vi "CmdWriter with Context.vi"() -> ()   [LabVIEW 2020]
doc: "Copyright © 2008 - 2024 VI Technologies B.V. \nALL RIGHTS RESERVED"
uses:
  <vilib>/dex/Stream Element Allocation Mode.ctl
  SuperNS/SuperNS.lvclass
  MsgData/MsgData.lvclass
panel:
  in  "Connection Config":T2={"BufferSize (100)"=100, "Connection Lost Timeout (2000 ms)"=2000, "Element Allocation Mode"=0, "Low latency mode"=enum."None (High througput mode)", "BG ConnCheck/Read period (200 ms)"=200, "OpenProcessWindow"=TRUE} {"Element Allocation Mode" items=["allocate as needed", "pre-allocate"]}
  out "error out":errorcluster
  in  "Remote EP Config":T3={"IP"="localhost", "Context"="ReadTestEnv", "Name"="ReaderTest"}
  in  "Local EP Config":cluster{"Context":string, "Name":string}={"Context"="WriteTestEnv", "Name"="WriterTest"}
  in  "Send":bool
  in  "Message":string
  # "Copyright (c) 2024, VI Technologies B.V.\nAll rights reserved.\n\nRedistribution and use in source and binary forms, with or without modification, are permitted provided that \nthe following conditions are met:\n\n * Redistributions of source code must retain the above copyright notice, this list of conditions and the \nfollowing disclaimer.\n * Redistributions in binary form must reproduce the above copyright notice, this list of conditions and the \nfollowing disclaimer in the documentation and/or other materials provided with the distribution.\n * Neither the name of VI Technologies B.V. nor the names of its contributors may be used to endorse or \npromote products derived from this software without specific prior written permission.\n\nTHIS SOFTWARE IS PROVIDED BY THE COPYRIGHT HOLDERS AND CONTRIBUTORS \"AS IS\" AND ANY EXPRESS OR \nIMPLIED WARRANTIES, INCLUDING, BUT NOT LIMITED TO, THE IMPLIED WARRANTIES OF MERCHANTABILITY \nAND FITNESS FOR A PARTICULAR PURPOSE ARE DISCLAIMED. IN NO EVENT SHALL THE COPYRIGHT OWNER OR \nCONTRIBUTORS BE LIABLE FOR ANY DIRECT, INDIRECT, INCIDENTAL, SPECIAL, EXEMPLARY, OR CONSEQUENTIAL \nDAMAGES (INCLUDING, BUT NOT LIMITED TO, PROCUREMENT OF SUBSTITUTE GOODS OR SERVICES; LOSS OF \nUSE, DATA, OR PROFITS; OR BUSINESS INTERRUPTION) HOWEVER CAUSED AND ON ANY THEORY OF LIABILITY, \nWHETHER IN CONTRACT, STRICT LIABILITY, OR TORT (INCLUDING NEGLIGENCE OR OTHERWISE) ARISING IN ANY \nWAY OUT OF THE USE OF THIS SOFTWARE, EVEN IF ADVISED OF THE POSSIBILITY OF SUCH DAMAGE.\n\nFor more information, please visit https://www.vi-tech.nl or contact us at info@vi-tech.nl"
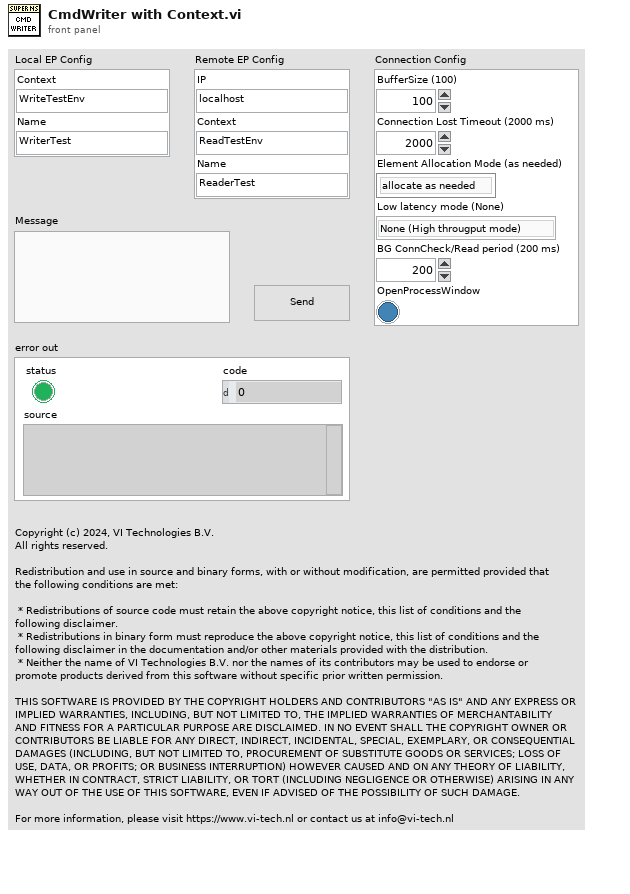
[diagram p1: front panel]
types:
  T1 = typedef "Stream Element Allocation Mode.ctl" = u32
  T2 = cluster{"BufferSize (100)":i32, "Connection Lost Timeout (2000 ms)":i32, "Element Allocation Mode":T1, "Low latency mode":enum16{"None (High througput mode)", "All Elements Read From Stream", "All Elements Available for Reading"}, "BG ConnCheck/Read period (200 ms)":i32, "OpenProcessWindow":bool}
  T3 = cluster{"IP":string, "Context":string, "Name":string}
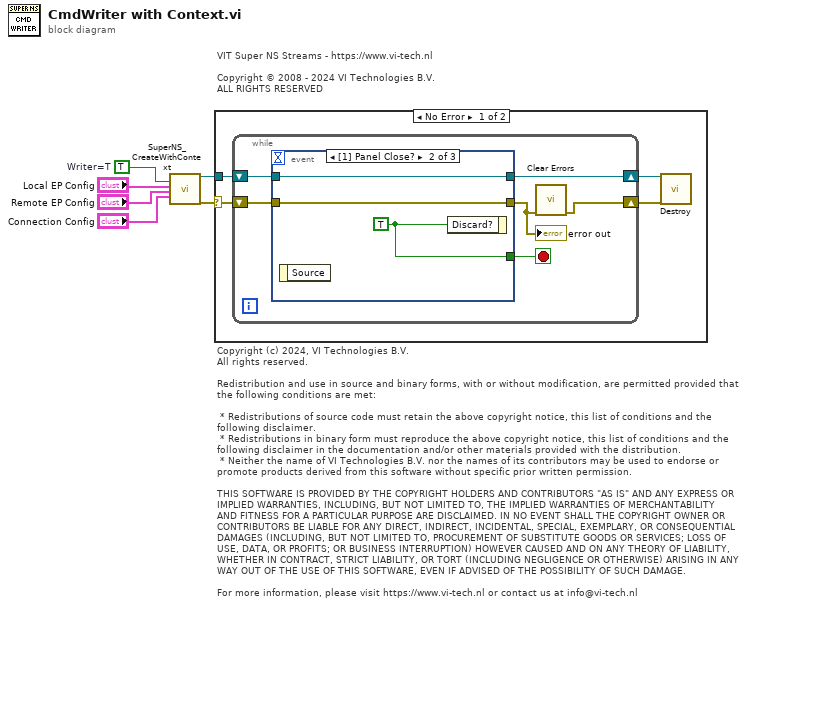
[diagram p0: block diagram]
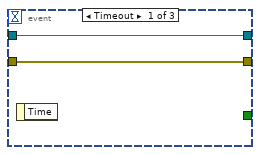
[diagram p2: hidden frame]
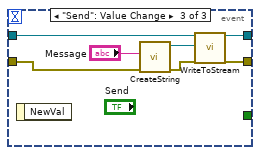
[diagram p3: hidden frame]
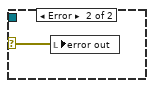
[diagram p4: hidden frame]
diagram:
  w4 = TRUE  # Writer=T
  # "VIT Super NS Streams - https://www.vi-tech.nl\n\nCopyright © 2008 - 2024 VI Technologies B.V. \nALL RIGHTS RESERVED"
  # "Copyright (c) 2024, VI Technologies B.V.\nAll rights reserved.\n\nRedistribution and use in source and binary forms, with or without modification, are permitted provided that \nthe following conditions are met:\n\n * Redistributions of source code must retain the above copyright notice, this list of conditions and the \nfollowing disclaimer.\n * Redistributions in binary form must reproduce the above copyright notice, this list of conditions and the \nfollowing disclaimer in the documentation and/or other materials provided with the distribution.\n * Neither the name of VI Technologies B.V. nor the names of its contributors may be used to endorse or \npromote products derived from this software without specific prior written permission.\n\nTHIS SOFTWARE IS PROVIDED BY THE COPYRIGHT HOLDERS AND CONTRIBUTORS \"AS IS\" AND ANY EXPRESS OR \nIMPLIED WARRANTIES, INCLUDING, BUT NOT LIMITED TO, THE IMPLIED WARRANTIES OF MERCHANTABILITY \nAND FITNESS FOR A PARTICULAR PURPOSE ARE DISCLAIMED. IN NO EVENT SHALL THE COPYRIGHT OWNER OR \nCONTRIBUTORS BE LIABLE FOR ANY DIRECT, INDIRECT, INCIDENTAL, SPECIAL, EXEMPLARY, OR CONSEQUENTIAL \nDAMAGES (INCLUDING, BUT NOT LIMITED TO, PROCUREMENT OF SUBSTITUTE GOODS OR SERVICES; LOSS OF \nUSE, DATA, OR PROFITS; OR BUSINESS INTERRUPTION) HOWEVER CAUSED AND ON ANY THEORY OF LIABILITY, \nWHETHER IN CONTRACT, STRICT LIABILITY, OR TORT (INCLUDING NEGLIGENCE OR OTHERWISE) ARISING IN ANY \nWAY OUT OF THE USE OF THIS SOFTWARE, EVEN IF ADVISED OF THE POSSIBILITY OF SUCH DAMAGE.\n\nFor more information, please visit https://www.vi-tech.nl or contact us at info@vi-tech.nl"
  n1 = call "SuperNS_CreateWithContext.vi"("Writer (F: Reader)"=w4, "Local EP Config"="Local EP Config", "Remote EP Config"="Remote EP Config", "Connection Config"="Connection Config") -> ("reference out"=w6:refnum<class "SuperNS.lvclass">, "error out"=w5:errorcluster)  [unwired: 14 in]
  n2 = case shown="No Error" w5 {
    selector: w5 -> [w7 w29]
    tunnel: w6 -> [w9 _]
    frame No Error {
      n3 = while {
        shift-right: [w14] -> w10
        shift-left: w9 -> [w15]
        shift-right: [w12] -> w8
        shift-left: w7 -> [w13]
        stop <- w16 stop-if-true
        n4 = event shown="[1] Panel Close?" {
          selector: _ -> [_ _ _]
          dyn-events: _ -> [_ _ _]
          timeout: _ -> [_ _ _]
          tunnel: [_ w21 _] -> w16
          tunnel: [w18 w20 w27] -> w14
          tunnel: w15 -> [w18 w20 w28]
          tunnel: w13 -> [w17 w19 w22]
          tunnel: [w17 w19 w26] -> w11
          event Timeout {
            n5 = event-data() -> ()  [unwired: 1 in, 1 out]
          }
          event Panel Close? {
            w21 = TRUE ("Discard?")
            n6 = event-data() -> ()  [unwired: 1 in, 1 out]
            n7 = event-data("Discard?"=w21) -> ()  [unwired: 1 in, 1 out]
          }
          event "Send": Value Change {
            n8 = event-data() -> ()  [unwired: 1 in, 1 out]
            n9 = call "CreateString.vi"("error in"=w22, "String"="Message") -> ("error out"=w23:errorcluster, "MsgData out"=w24:refnum<class "MsgData.lvclass">)  [unwired: 8 in]
            n10 = call-dynamic "WriteToStream.vi"("reference in"=w28, "LabVIEW Object"=w24, "error in"=w23) -> ("reference out"=w27:refnum<class "SuperNS.lvclass">, "error out"=w26:errorcluster)  [unwired: 14 in, 1 out]
          }
        }
        "error out" <- w11
        n11 = call <vilib>:"Clear Errors.vi"("error in (no error)"=w11) -> ("error out"=w12:errorcluster)  [unwired: 5 in, 1 out]
      }
      n12 = call-dynamic "Destroy.vi"("reference in"=w10, "error in (no error)"=w8) -> ()  [unwired: 16 in, 2 out]
    }
    frame Error {
      n13 = local write "error out"(w29) -> ()
    }
  }
